vi "checkSamplingRates.vi"(8 "error in (no error)":errorcluster, 11 "Available Sigals in":refnum<class "ISignal.lvclass">[](array[class])) -> (0 "error out":errorcluster, 1 "SampleRate":dbl, 2 "Boolean":bool, 3 "Array":refnum<class "ISignal.lvclass">[](array[class]))   [LabVIEW 2022 SP3, in "StreamReader.lvlib"]
uses:
  <instrlib>/openDAQ/Examples/StreamReader/StreamReader.lvlib
  <instrlib>/openDAQ/Public/Classes/ISignal/ISignal.lvclass
  <instrlib>/openDAQ/Public/Classes/IBaseObject/Polymorphic/queryInterface/queryNumberInterface.vi
  <instrlib>/openDAQ/Public/Classes/IDataDescriptor/IDataDescriptor.lvclass
  <instrlib>/openDAQ/Public/Classes/IDataRule/IDataRule.lvclass
  <instrlib>/openDAQ/Public/Classes/daqCoreTypes/IRatio/IRatio.lvclass
  <instrlib>/openDAQ/Public/Classes/daqCoreTypes/IDict/IDict.lvclass
  <instrlib>/openDAQ/Public/Classes/IBaseObject/IBaseObject.lvclass
  <instrlib>/openDAQ/Public/Classes/daqCoreTypes/INumber/INumber.lvclass
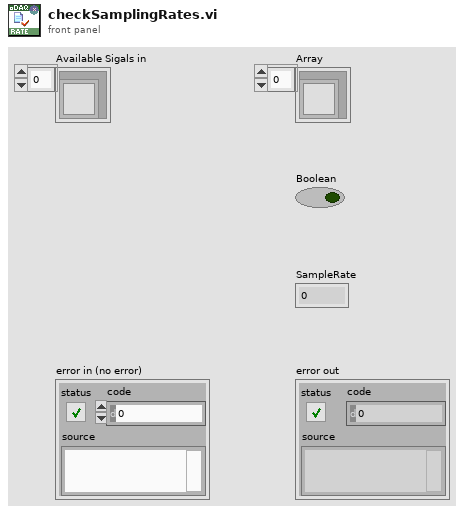
[diagram p1: front panel]
types:
  T1 = typedef "openDAQ.lvlib/IBaseObject.lvlib/IDataRule.lvlib/IDataRule.lvclass/DataRuleType.ctl" = u16
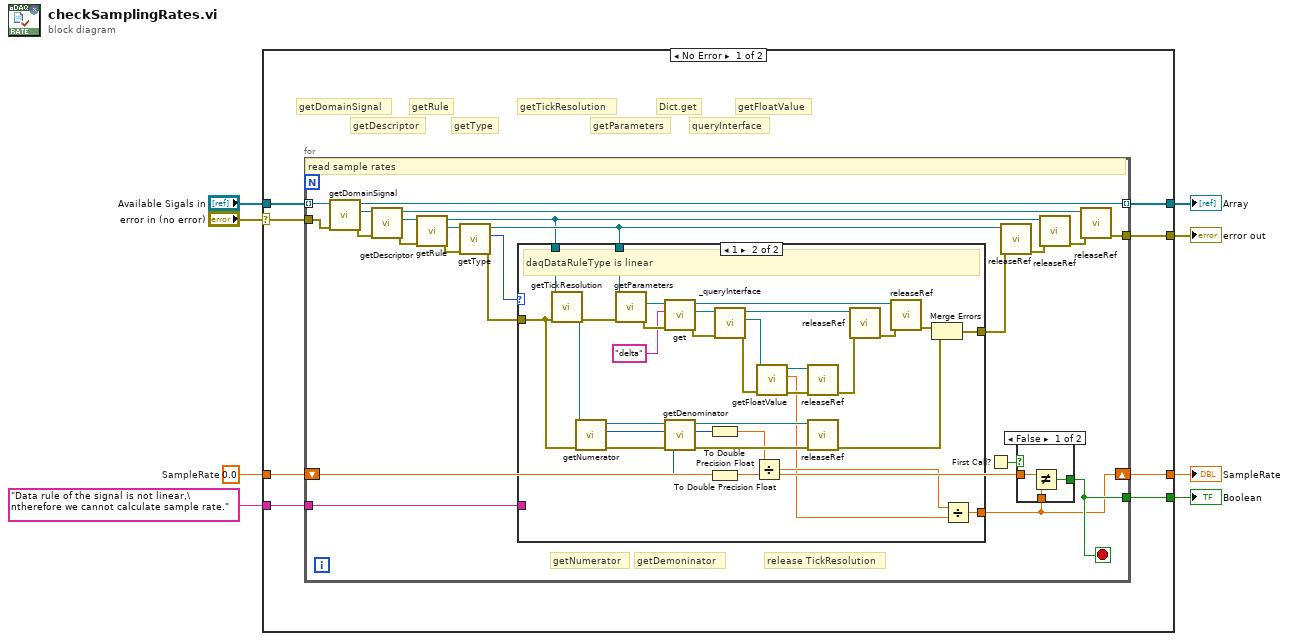
[diagram p0: block diagram]
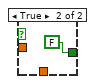
[diagram p2: hidden frame]
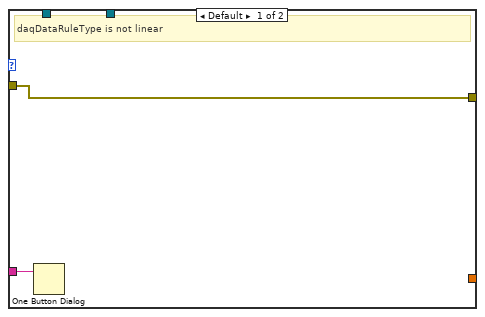
[diagram p3: hidden frame]
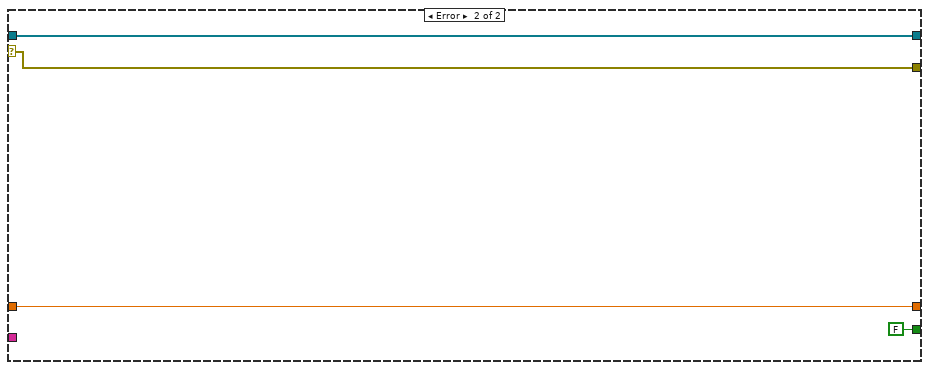
[diagram p4: hidden frame]
diagram:
  w3 = 0.0  # SampleRate
  n1 = case shown="No Error" "error in (no error)" {
    selector: "error in (no error)" -> [w9 w80]
    tunnel: [w16 w81] -> w8
    tunnel: [w15 w79] -> w7
    tunnel: "Data rule of the signal is not linear,\ntherefore we cannot calculate sample rate." ("modulePath") -> [w14 _]
    tunnel: [w13 FALSE] -> w5
    tunnel: [w12 w80] -> w4
    tunnel: w3 -> [w11 w79]
    tunnel: "Available Sigals in" -> [w10 w81]
    frame No Error {
      # "getFloatValue"
      # "queryInterface"
      # "Dict.get"
      # "getParameters"
      # "getTickResolution"
      # "getType"
      # "getRule"
      # "getDescriptor"
      # "getDomainSignal"
      n2 = for {
        tunnel: w10 -> [w22] mode=indexing
        tunnel: [w26] -> w12
        tunnel: w9 -> [w39]
        tunnel: w14 -> [w29]
        tunnel: [w21] -> w16 mode=indexing
        shift-right: [w17] -> w15
        shift-left: w11 -> [w20]
        tunnel: [w19] -> w13
        stop <- w19 stop-if-true
        # "release TickResolution"
        # "getDemoninator"
        # "getNumerator"
        # "read sample rates"
        n3 = call <instrlib>:"getDomainSignal.vi"("error in (no error)"=w39, "ISignal in"=w22) -> ("error out"=w23:errorcluster, "DomainSignal out"=w38:refnum<class "ISignal.lvclass">, "ISignal out"=w21:refnum<class "ISignal.lvclass">)  [unwired: 7 in]
        n4 = call <instrlib>:"getDescriptor.vi"("error in (no error)"=w23, "ISignal in"=w38) -> ("error out"=w24:errorcluster, "DataDescriptor out"=w25:refnum<class "IDataDescriptor.lvclass">, "ISignal out"=w28:refnum<class "ISignal.lvclass">)  [unwired: 7 in]
        n5 = call <instrlib>:"getRule.vi"("error in (no error)"=w24, "IDataDescriptor in"=w25) -> ("error out"=w34:errorcluster, "DataRule out"=w35:refnum<class "IDataRule.lvclass">, "IDataDescriptor out"=w27:refnum<class "IDataDescriptor.lvclass">)  [unwired: 7 in]
        n6 = call <instrlib>:"getType.vi"("error in (no error)"=w34, "IDataRule in"=w35) -> ("error out"=w32:errorcluster, "DataRuleType"=w33:T1, "IDataRule out"=w31:refnum<class "IDataRule.lvclass">)  [unwired: 7 in]
        n7 = case shown="1" w33 {
          tunnel: w29 -> [w45 _]
          tunnel: w32 -> [w44 w62]
          tunnel: w27 -> [_ w74]
          tunnel: w31 -> [_ w72]
          tunnel: [w44 w53] -> w30
          tunnel: [_ w52] -> w17
          frame Default {
            # "daqDataRuleType is not linear"
            n8 = One Button Dialog(message=w45) -> ()  [unwired: 1 in, 1 out]
          }
          frame 1 {
            # "daqDataRuleType is linear"
            n9 = call <instrlib>:"getTickResolution.vi"("error in (no error)"=w62, "IDataDescriptor in"=w74) -> ("error out"=w73:errorcluster, "TickResolution out"=w64:refnum<class "IRatio.lvclass">)  [unwired: 7 in, 1 out]
            n10 = call <instrlib>:"getNumerator.vi"("error in (no error)"=w62, "IRatio in"=w64) -> ("error out"=w61:errorcluster, "Numerator out"=w58:i64, "IRatio out"=w63:refnum<class "IRatio.lvclass">)  [unwired: 7 in]
            n11 = call <instrlib>:"getParameters.vi"("error in (no error)"=w73, "IDataRule in"=w72) -> ("error out"=w51:errorcluster, "Parameters out"=w71:refnum<class "IDict.lvclass">)  [unwired: 7 in, 1 out]
            n12 = call <instrlib>:"get.vi"("error in (no error)"=w51, "Key in"="delta" ("String"), "IDict in"=w71) -> ("error out"=w48:errorcluster, "Value out"=w50:refnum<class "IBaseObject.lvclass">, "IDict out"=w56:refnum<class "IDict.lvclass">)  [unwired: 6 in]
            n13 = call <instrlib>:"getDenominator.vi"("error in (no error)"=w61, "IRatio in"=w63) -> ("error out"=w75:errorcluster, "Denominator out"=w60:i64, "IRatio out"=w76:refnum<class "IRatio.lvclass">)  [unwired: 7 in]
            n14 = To Double Precision Float(number=w60) -> (double precision float=w59:dbl)
            n15 = To Double Precision Float(number=w58) -> (double precision float=w57:dbl)
            n16 = call-poly <instrlib>:"_queryInterface.vi"("error in (no error)"=w48, "IBaseObject in"=w50) -> ("error out"=w70:errorcluster, "INumber out"=w66:refnum<class "INumber.lvclass">, "IBaseObject out"=w65:refnum<class "IBaseObject.lvclass">)  [unwired: 7 in]
            n17 = Divide(x=w59, y=w57) -> (x/y=w47:dbl)
            n18 = call <instrlib>:"getFloatValue.vi"("error in (no error)"=w70, "INumber in"=w66) -> ("error out"=w68:errorcluster, "Float Value out"=w46:dbl, "INumber out"=w69:refnum<class "INumber.lvclass">)  [unwired: 7 in]
            n19 = call-dynamic "releaseRef.vi"("error in (no error)"=w68, "IBaseObject in"=w69) -> ("error out"=w67:errorcluster)  [unwired: 9 in]
            n20 = call-dynamic "releaseRef.vi"("error in (no error)"=w75, "IBaseObject in"=w76) -> ("error out"=w77:errorcluster)  [unwired: 9 in]
            n21 = call-dynamic "releaseRef.vi"("error in (no error)"=w67, "IBaseObject in"=w65) -> ("error out"=w55:errorcluster)  [unwired: 9 in]
            n22 = call-dynamic "releaseRef.vi"("error in (no error)"=w55, "IBaseObject in"=w56) -> ("error out"=w54:errorcluster)  [unwired: 9 in]
            n23 = Merge Errors(w54, w77) -> (w53:errorcluster)
            n24 = Divide(x=w47, y=w46) -> (x/y=w52:dbl)
          }
        }
        n25 = First Call?() -> (First Call?: T/F=w18:bool)
        n26 = call-dynamic "releaseRef.vi"("error in (no error)"=w30, "IBaseObject in"=w31) -> ("error out"=w36:errorcluster)  [unwired: 9 in]
        n27 = case shown="False" w18 {
          tunnel: w20 -> [w41 _]
          tunnel: [w42 FALSE] -> w19
          tunnel: w17 -> [w40 _]
          frame False {
            n28 = Not Equal?(x=w41, y=w40) -> (x != y?=w42:bool)
          }
          frame True {
          }
        }
        n29 = call-dynamic "releaseRef.vi"("error in (no error)"=w36, "IBaseObject in"=w27) -> ("error out"=w37:errorcluster)  [unwired: 9 in]
        n30 = call-dynamic "releaseRef.vi"("error in (no error)"=w37, "IBaseObject in"=w28) -> ("error out"=w26:errorcluster)  [unwired: 9 in]
      }
    }
    frame Error {
    }
  }
  "Array" <- w8
  "SampleRate" <- w7
  "Boolean" <- w5
  "error out" <- w4
